vi "FPGA Phasor Measurement.vi"(0 "resampled data":T4, 1 "number of channels":T3=1 items=["1"=1, "2"=2, "3"=3, "4"=4, "5"=5, "6"=6, "7"=7, "8"=8, "9"=9, "10"=10, "11"=11, "12"=12, "13"=13, "14"=14, "15"=15, "16"=16], 5 "resampling info":T1={"nominal frequency"=enum."50 Hz", "resampling valid?"=FALSE, "samples per cycle"=192}, 9 "input valid? (T)":bool=TRUE, 12 "ready for output? (T)":bool=TRUE) -> (4 "output data":T2 {"timestamp [s]" format="%#.6g"; "phase [pi]" format="%#.6g"}, 10 "output valid?":bool, 14 "ready for input?":bool, 15 "error":i32)   [LabVIEW 2013, in "NI_EP_PMU_FPGA.lvlib"]
doc: "LabVIEW no longer supports this VI. Use the FPGA Phasor Measurement for M Class VI or the FPGA Phasor Measurement for P Class VI instead.\n\nComputes the instantaneous magnitude, phase, and frequency values of the fundamental frequency component, at an output rate of 24 samples per cycle. You must use the FPGA Resampling VI to resample even-time-spaced voltage and current signals into even-angle-spaced signals before running this VI."
uses:
  <vilib>/addons/Electrical Power/PMU/NI_EP_PMU_FPGA.lvlib
  <vilib>/addons/Electrical Power/PQ/Resampling/FPGA/subVIs/fpga_Resampled.ctl
  <vilib>/addons/Electrical Power/PQ/Resampling/FPGA/subVIs/fpga_NofCH.ctl
  <vilib>/addons/Electrical Power/PMU/FPGA/subVIs/fpga_OutputDataType.ctl
  <vilib>/addons/Electrical Power/PQ/Resampling/FPGA/subVIs/fpga_Resampling Info.ctl
  <vilib>/addons/Electrical Power/PQ/Resampling/NI_EP_Resample_FPGA.lvlib
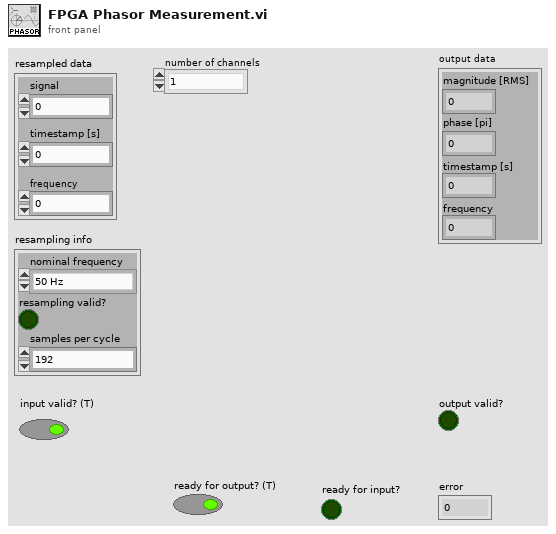
[diagram p1: front panel]
types:
  T1 = typedef "NI_EP_Resample_FPGA.lvlib/fpga_Resampling Info.ctl" = cluster{"nominal frequency":enum16{"50 Hz", "60 Hz"}, "resampling valid?":bool, "samples per cycle":u16}
  T2 = typedef "NI_EP_PMU_FPGA.lvlib/fpga_OutputDataType.ctl" = cluster{"magnitude [RMS]":fxp<+,32,6>, "phase [pi]":fxp<+/-,32,2>, "timestamp [s]":fxp<+,64,32>, "frequency":fxp<+,32,8>}
  T3 = typedef "NI_EP_Resample_FPGA.lvlib/fpga_NofCH.ctl" = u8
  T4 = typedef "NI_EP_Resample_FPGA.lvlib/fpga_Resampled.ctl" = cluster{"signal":fxp<+/-,32,3>, "timestamp [s]":fxp<+,64,32>, "frequency":fxp<+,32,8>}
  T5 = cluster{"rms magnitude":fxp<+,32,6>, "phase":fxp<+/-,32,2>, "Time Stamp out":fxp<+,64,32>, "Frequency output":fxp<+,32,8>}
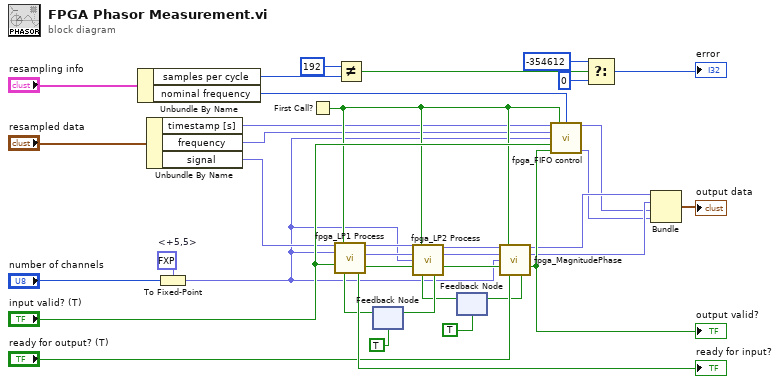
[diagram p0: block diagram]
diagram:
  w13 = fxp<+,5,5> 0.0  # <+5,5>
  n1 = Unbundle By Name("resampling info") -> ("samples per cycle"=w6:u16, "nominal frequency"=w7:enum16{"50 Hz", "60 Hz"})
  n2 = Unbundle By Name("resampled data") -> ("timestamp [s]"=w16:fxp<+,64,32>, "frequency"=w14:fxp<+,32,8>, "signal"=w15:fxp<+/-,32,3>)
  n3 = To Fixed-Point(fixed-point type=w13, number="number of channels") -> (fixed-point=w12:fxp<+,5,5>)
  n4 = First Call?() -> (First Call?: T/F=w17:bool)
  n5 = Not Equal?(x=u16 192, y=w6) -> (x != y?=w4:bool)
  n6 = feedback #1(TRUE ("ready for input")) -> (w26:bool)
  n7 = call <vilib>:"fpga_LP1 Process.vi"("input data"=w15, "reset"=w17, "Ch"=w12, "input valid"="input valid? (T)", "ready for output"=w26) -> ("re"=w29:fxp<+/-,32,5>, "im"=w28:fxp<+/-,32,5>, "output valid"=w25:bool, "ready for input"=→"ready for input?":bool)  [unwired: 7 in]
  n8 = feedback #2(TRUE ("ready for input")) -> (w19:bool)
  n9 = call <vilib>:"fpga_LP2 Process.vi"("re"=w29, "reset"=w17, "im"=w28, "#Ch"=w12, "input valid"=w25, "ready for output"=w19) -> ("re filtered"=w23:fxp<+/-,32,6>, "im filtered"=w22:fxp<+/-,32,6>, "output valid"=w21:bool, "ready for input"=w27:bool)  [unwired: 6 in]
  n10 = feedback-in #1(w27) -> ()
  n11 = call <vilib>:"fpga_MagnitudePhase.vi"("re"=w23, "reset"=w17, "im"=w22, "Ch"=w12, "input valid"=w21, "ready for output"="ready for output? (T)") -> ("rms magnitude"=w11:fxp<+,32,6>, "phase"=w10:fxp<+/-,32,2>, "output valid"=w34:bool, "ready for input"=w20:bool)  [unwired: 6 in]
  "output valid?" <- w34
  n12 = feedback-in #2(w20) -> ()
  n13 = call <vilib>:"fpga_FIFO control.vi"("Time stamp"=w16, "reset"=w17, "nominal frequency"=w7, "Frequency"=w14, "#ch"=w12, "PMU VI input valid"="input valid? (T)", "PMU VI output valid"=w34) -> ("Time Stamp out"=w9:fxp<+,64,32>, "Frequency output"=w8:fxp<+,32,8>)  [unwired: 7 in]
  n14 = Select(t=-354612 ("error"), s=w4, f=0) -> (s? t:f=→"error":i32)
  n15 = Bundle("rms magnitude"=w11, "phase"=w10, "Time Stamp out"=w9, "Frequency output"=w8) -> (→"output data":T5)  [unwired: 1 in]
